vi "Ardwino-decifer-return.vi"(5 "Log file path":path=path "C:/Users/gsfcprime/Documents/Logs/FW_test-logs", 6 "New file?":bool, 7 "Reset history":bool, 8 "cycle  time":dbl, 9 "Switch query response":string, 10 "Responses history 2D in":string[][](array[string])=[["[Command Recv(18)]", "Motor ID     :", "State        :", "Direction    :", "Switch       :", "# of steps   :", "Step max rate:", "Ramp Slope   :", "# of position:", "com_success", "Q1S", "EOR1:"]], 11 "Arduino Response":string) -> (1 "Waveform Graph":dbl[][](graph), 2 "Responses history 2D out":string[][](array[string])=[["[Command Recv(18)]", "Motor ID     :", "State        :", "Direction    :", "Switch       :", "# of steps   :", "Step max rate:", "Ramp Slope   :", "# of position:", "com_success", "Q1S", "EOR1:"]], 3 "New  string to append":string[](array[string])=["[Command Recv(18)]", "Motor ID     :", "State        :", "Direction    :", "Switch       :", "# of steps   :", "Step max rate:", "Ramp Slope   :", "# of position:", "com_success", "Q1S", "EOR1:"], 4 "Log file out":path=path "C:/Users/gsfcprime/Documents/PRIME_documentation/FW_test_logs")   [LabVIEW 2021]
uses:
  <vilib>/Utility/file.llb/Write Delimited Spreadsheet (string).vi
  <vilib>/regexp/Match Regular Expression.xnode
panel:
  in  "(col) 2":i32=13
  out "Sw stae":u32(colorbox) caption="Sw state"
  out "after match":string
  out "before match":string
  out "m":i32
  out "substring":string
  in  "Motor #":string="0"
  in  "(col)":i32=12
  out "Array":dbl[](array[numeric])
  in  "List parameters":string[](array[string])=["[Command Recv(18)]", "Motor ID     :", "State        :", "Direction    :", "Switch       :", "# of steps   :", "Step max rate:", "Ramp Slope   :", "# of position:", "com_success", "Q1S", "EOR1:"]
  out "Ardwino responses -  Array":string[](array[string])=["[Command Recv(18)]", "Motor ID     :", "State        :", "Direction    :", "Switch       :", "# of steps   :", "Step max rate:", "Ramp Slope   :", "# of position:", "com_success", "Q1S", "EOR1:"]
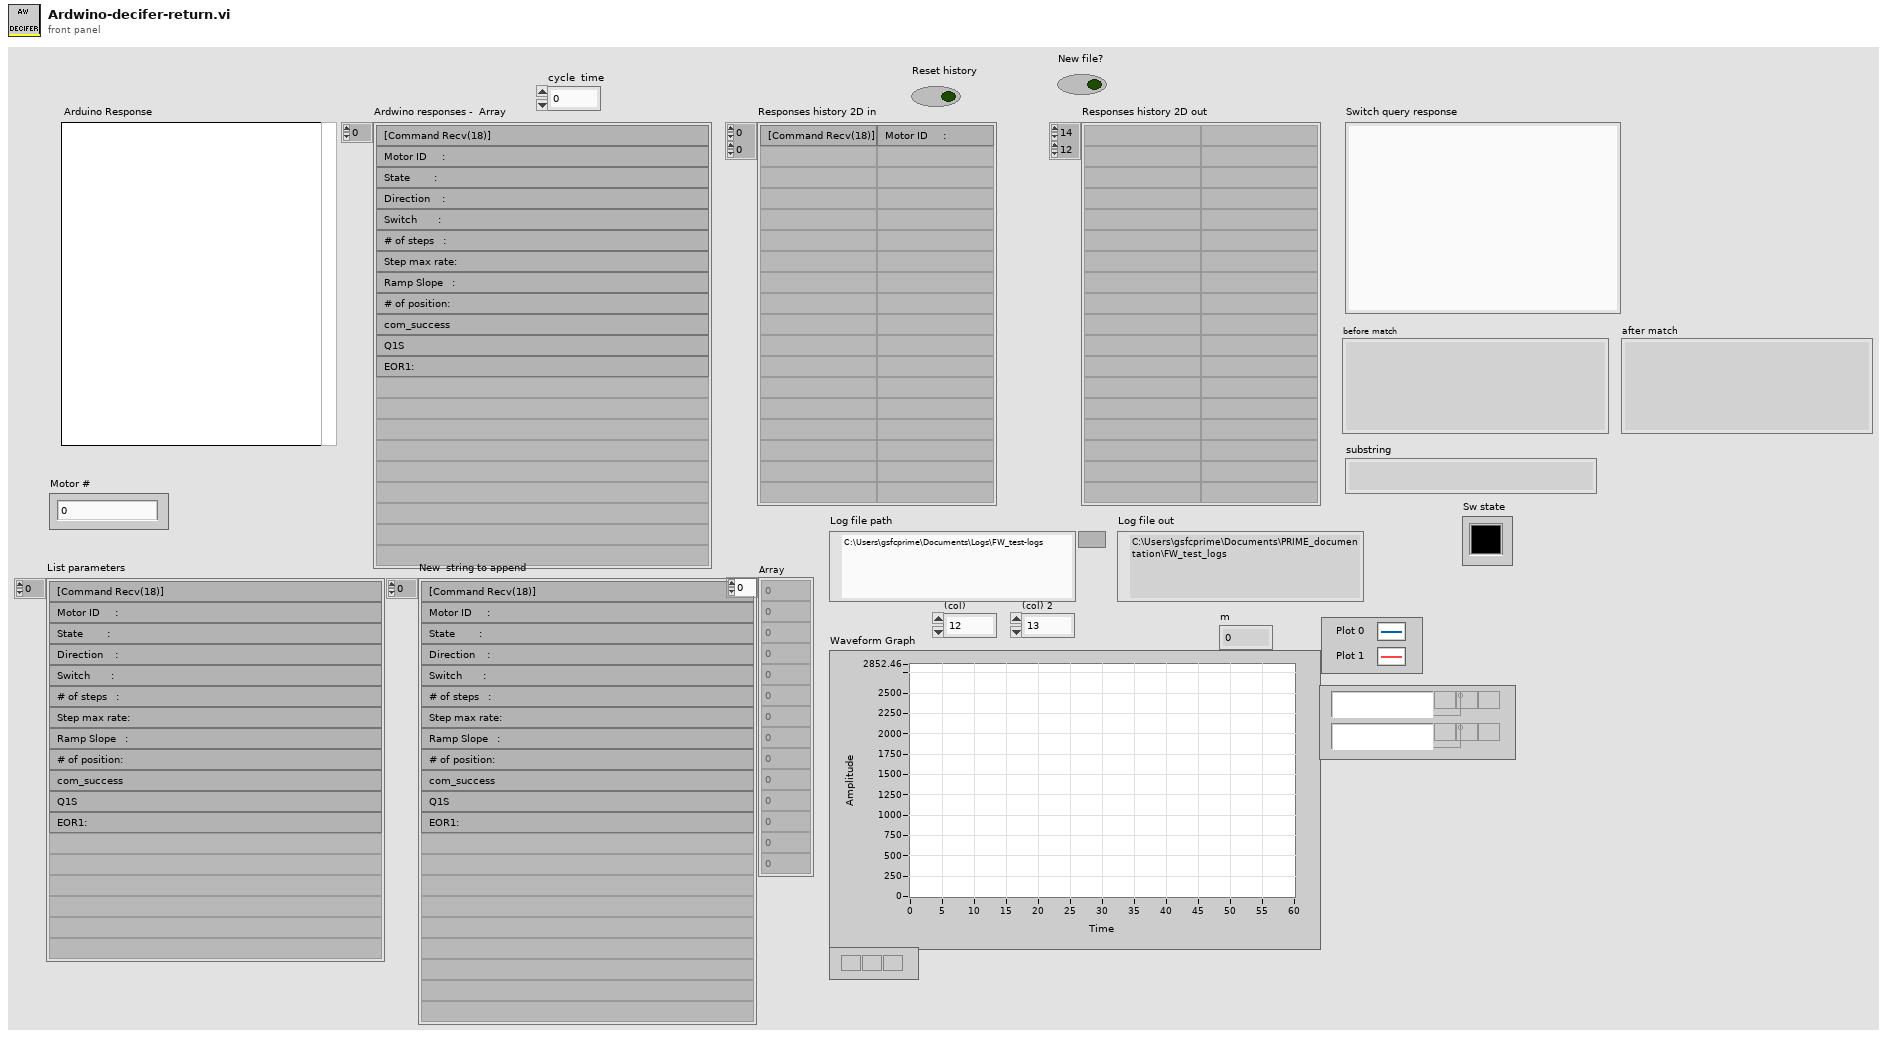
[diagram p1: front panel]
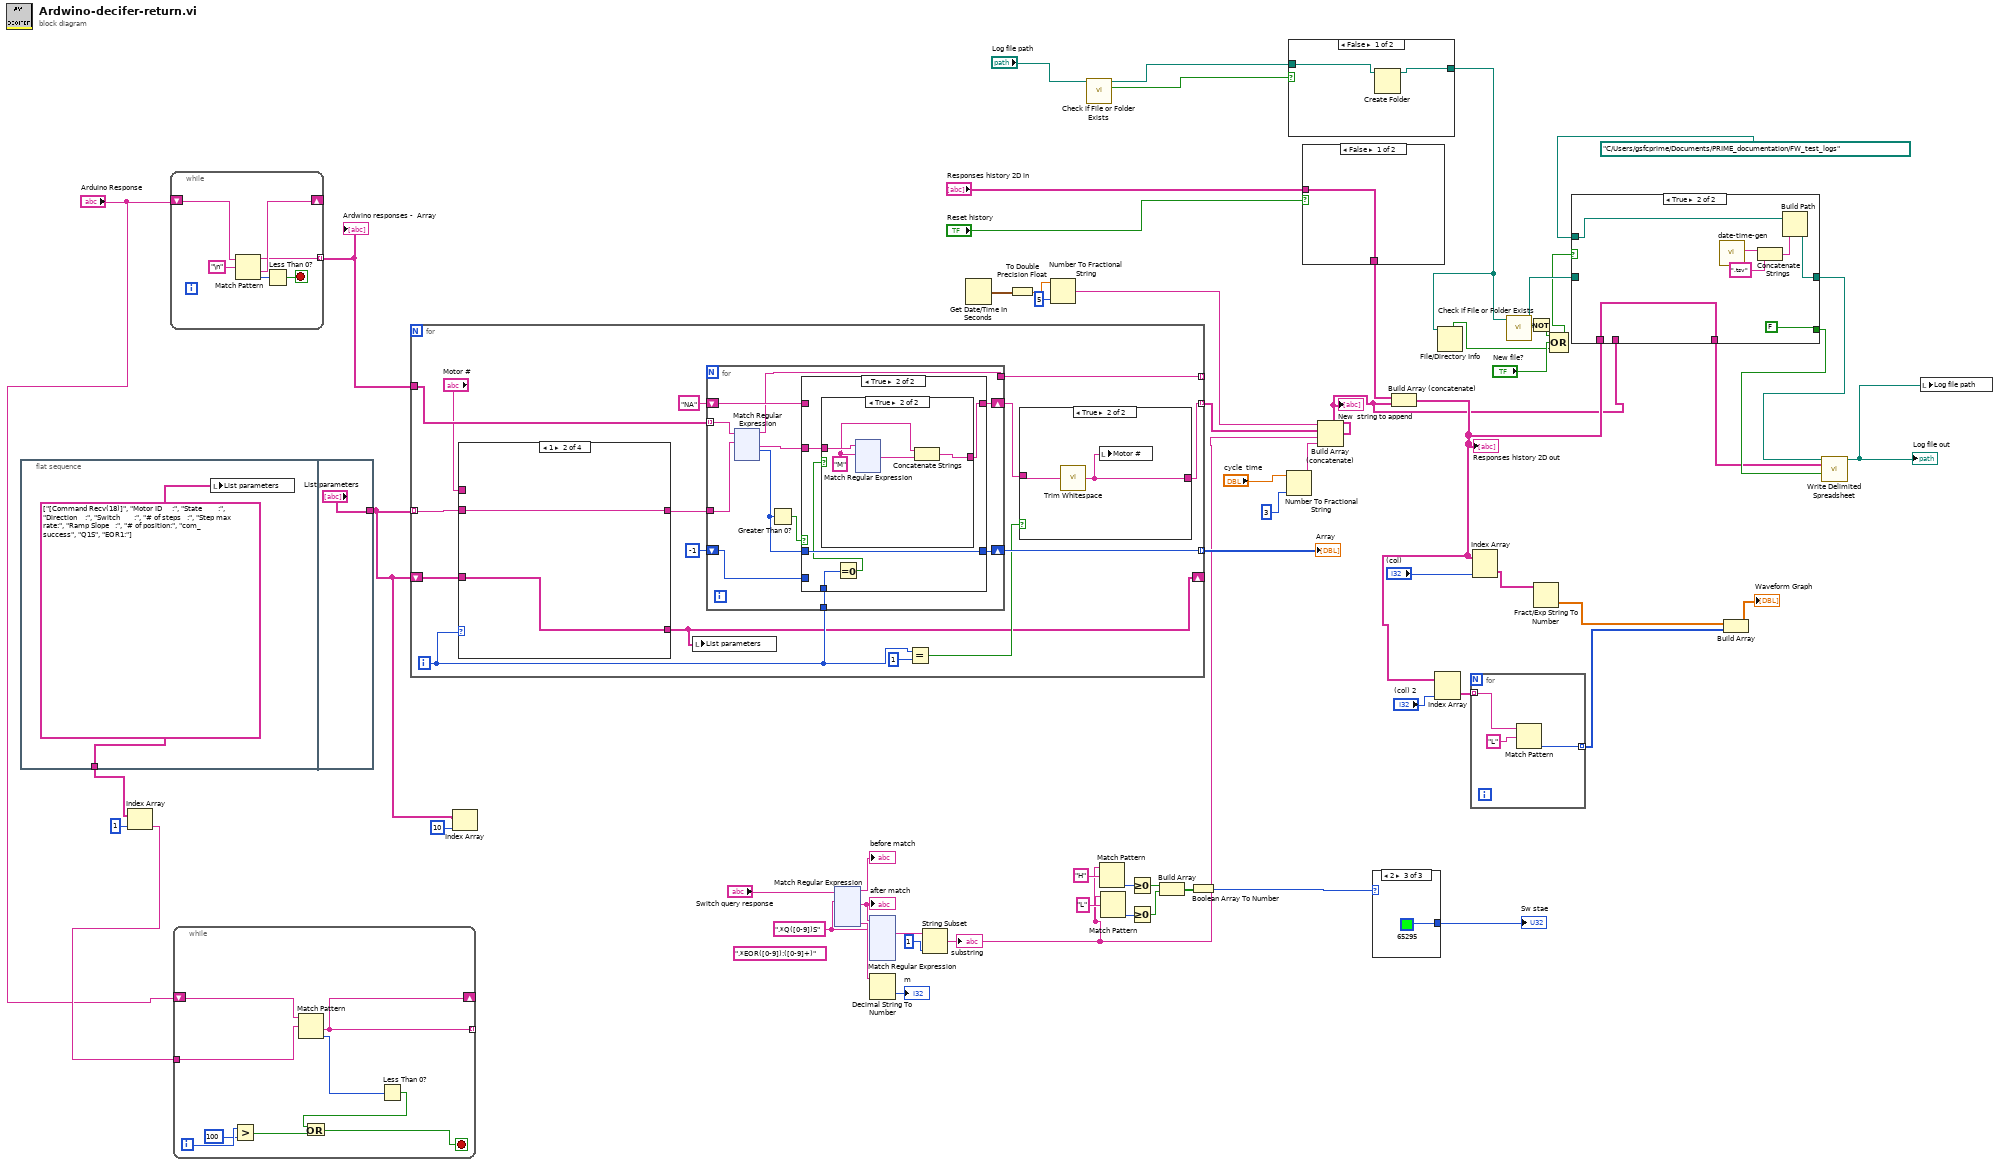
[diagram p0: block diagram]
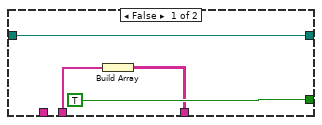
[diagram p3: hidden frame]
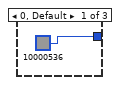
[diagram p4: hidden frame]
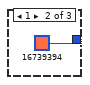
[diagram p5: hidden frame]
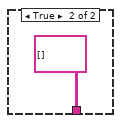
[diagram p6: hidden frame]
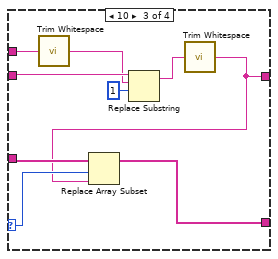
[diagram p8: hidden frame]
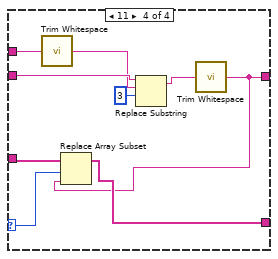
[diagram p9: hidden frame]
diagram:
  w43 = ".*Q([0-9])S" ("regular expression")
  (unwired) ".*EOR([0-9]):([0-9]+)" ("regular expression")
  n1 = flat-sequence {
    tunnel: [w62] -> w51
    tunnel: ["List parameters"] -> w55
    frame #0 {
      w62 = string[] ["[Command Recv(18)]", "Motor ID     :", "State        :", "Direction    :", "Switch       :", "# of steps   :", "Step max rate:", "Ramp Slope   :", "# of position:", "com_success", "Q1S", "EOR1:"] ("List parameters")
      n2 = local write "List parameters"(w62) -> ()
    }
    frame #1 {
    }
  }
  n3 = Index Array(array=w51, index=1) -> (element=w49:string)
  n4 = while {
    shift-right: [w68] -> _
    shift-left: "Arduino Response" -> [w69]
    tunnel: [w65] -> w52 mode=indexing
    stop <- w66 stop-if-true
    n5 = Match Pattern(string=w69, regular expression="\n") -> (before substring=w65:string, after substring=w68:string, offset past match=w67:i32)  [unwired: 1 in, 1 out]
    n6 = Less Than 0?(x=w67) -> (x < 0?=w66:bool)
  }
  "Ardwino responses -  Array" <- w52
  n7 = while {
    tunnel: w49 -> [w78]
    tunnel: [w75] -> _ mode=indexing
    shift-right: [w75] -> _
    shift-left: "Arduino Response" -> [w76]
    i -> [w73]
    stop <- w70 stop-if-true
    n8 = Greater?(x=w73, y=100) -> (0:w71:bool)
    n9 = Match Pattern(string=w76, regular expression=w78) -> (after substring=w75:string, offset past match=w77:i32)  [unwired: 1 in, 2 out]
    n10 = Less Than 0?(x=w77) -> (x < 0?=w74:bool)
    n11 = Or(x=w74, y=w71) -> (x .or. y?=w70:bool)
  }
  n12 = for {
    tunnel: w55 -> [w84] mode=indexing
    tunnel: w52 -> [w93]
    tunnel: [w81] -> w53 mode=indexing
    tunnel: [w90] -> w61 mode=indexing
    tunnel: [w89] -> _ mode=indexing
    shift-right: [w79] -> _
    shift-left: w55 -> [w80]
    i -> [w85]
    n13 = case shown="1" w85 {
      selector: w85 -> [_ _ w100 w111]
      tunnel: w84 -> [w95 w97 w106 w114]
      tunnel: "Motor #" -> [_ _ w105 w108]
      tunnel: [w95 w97 w98 w109] -> w82
      tunnel: w80 -> [w94 w96 w102 w113]
      tunnel: [w94 w96 w101 w112] -> w79
      frame 0, Default {
      }
      frame 1 {
      }
      frame 10 {
        n14 = call <vilib>:"Trim Whitespace.vi"("string"=w105) -> ("trimmed string"=w103:string)  [unwired: 1 in]
        n15 = Replace Substring(3:1 ("offset (0)"), 4:w103, 5:w106) -> (1:w99:string)  [unwired: 1 in, 1 out]
        n16 = call <vilib>:"Trim Whitespace.vi"("string"=w99) -> ("trimmed string"=w98:string)  [unwired: 1 in]
        n17 = Replace Array Subset(array=w102, new element=w98, index=w100) -> (w101:string[])
      }
      frame 11 {
        n18 = call <vilib>:"Trim Whitespace.vi"("string"=w108) -> ("trimmed string"=w107:string)  [unwired: 1 in]
        n19 = Replace Substring(3:3 ("offset (0)"), 4:w107, 5:w114) -> (1:w110:string)  [unwired: 1 in, 1 out]
        n20 = call <vilib>:"Trim Whitespace.vi"("string"=w110) -> ("trimmed string"=w109:string)  [unwired: 1 in]
        n21 = Replace Array Subset(array=w113, new element=w109, index=w111) -> (w112:string[])
      }
    }
    n22 = local write "List parameters"(w79) -> ()
    n23 = for {
      tunnel: w93 -> [w123] mode=indexing
      tunnel: w82 -> [w129]
      shift-right: [w121] -> w90
      shift-left: -1 ("offset past match") -> [w128]
      shift-right: [w127] -> w86
      shift-left: "NA" ("Arduino Responses") -> [w126]
      tunnel: [w120] -> w89
      tunnel: w85 -> [w119]
      n24 = xnode "Match Regular Expression"("input string"=w123, "regular expression"=w129) -> ("before match"=w120:string, "after match"=w125:string, "offset past match"=w122:i32)  [unwired: 4 in, 2 out]
      n25 = Greater Than 0?(x=w122) -> (x > 0?=w124:bool)
      n26 = case shown="True" w124 {
        tunnel: w128 -> [w247 _]
        tunnel: [w248 w249] -> w127
        tunnel: w126 -> [w248 _]
        tunnel: w125 -> [_ w250]
        tunnel: w122 -> [_ w253]
        tunnel: [w247 w253] -> w121
        tunnel: w119 -> [_ w252]
        frame False {
        }
        frame True {
          n27 = Equal To 0?(x=w252) -> (x = 0?=w251:bool)
          n28 = case shown="True" w251 {
            tunnel: w250 -> [w254 w258]
            tunnel: [w254 w256] -> w249
            frame False {
            }
            frame True {
              w255 = "M" ("regular expression")
              n29 = xnode "Match Regular Expression"("input string"=w258, "regular expression"=w255) -> ("after match"=w257:string)  [unwired: 4 in, 4 out]
              n30 = Concatenate Strings(w255, w257) -> (w256:string)
            }
          }
        }
      }
    }
    n31 = Equal?(x=w85, y=1) -> (x = y?=w87:bool)
    n32 = case shown="True" w87 {
      tunnel: w86 -> [w116 w118]
      tunnel: [w116 w117] -> w81
      frame False {
      }
      frame True {
        n33 = call <vilib>:"Trim Whitespace.vi"("string"=w118) -> ("trimmed string"=w117:string)  [unwired: 1 in]
        n34 = local write "Motor #"(w117) -> ()
      }
    }
  }
  "Array" <- w61
  n35 = Index Array(array=w55, index=10) -> ()  [unwired: 1 out]
  n36 = xnode "Match Regular Expression"("input string"="Switch query response", "regular expression"=w43) -> ("before match"=→"before match":string, "after match"=w44:string, "submatch 1"=w47:string)  [unwired: 4 in, 3 out]
  "after match" <- w44
  n37 = xnode "Match Regular Expression"("input string"=w44, "regular expression"=w43) -> ("after match"=w42:string)  [unwired: 4 in, 6 out]
  n38 = Decimal String To Number(string=w47) -> (number=→"m":i32)  [unwired: 2 in, 1 out]
  n39 = String Subset(string=w42, length (rest)=1 ("length (rest)")) -> (substring=w37:string)  [unwired: 1 in]
  "substring" <- w37
  n40 = Get Date/Time In Seconds() -> (seconds since 1Jan1904=w17:timestamp)
  n41 = To Double Precision Float(number=w17) -> (double precision float=w14:dbl)
  n42 = Number To Fractional String(number=w14, precision (6)=i16 5) -> (F-format string=w15:string)  [unwired: 2 in]
  n43 = call <vilib>:"Check if File or Folder Exists.vi"("path"="Log file path") -> ("file or folder exists?"=w4:bool, "dup path"=w5:path)  [unwired: 8 in, 1 out]
  n44 = Match Pattern(string=w37, regular expression="H") -> (offset past match=w36:i32)  [unwired: 1 in, 3 out]
  n45 = Match Pattern(string=w37, regular expression="L") -> (offset past match=w35:i32)  [unwired: 1 in, 3 out]
  n46 = Greater Or Equal To 0?(x=w36) -> (x >= 0?=w33:bool)
  n47 = Greater Or Equal To 0?(x=w35) -> (x >= 0?=w34:bool)
  n48 = Build Array(w33, w34) -> (w32:bool[])
  n49 = Boolean Array To Number(Boolean array=w32) -> (number=w31:u32)
  n50 = Number To Fractional String(number="cycle  time", precision (6)=i16 3) -> (F-format string=w1:string)  [unwired: 2 in]
  n51 = case shown="False" w4 {
    tunnel: w5 -> [w377 w378]
    tunnel: [w376 w378] -> w6
    frame False {
      n52 = Create Folder(path (use dialog)=w377) -> (created path=w376:path)  [unwired: 2 in, 2 out]
    }
    frame True {
    }
  }
  n53 = case shown="False" "Reset history" {
    tunnel: "Responses history 2D in" -> [w379 _]
    tunnel: [w379 string[][] [] ("Responses history 2D in")] -> w59
    frame False {
    }
    frame True {
    }
  }
  n54 = Build Array (concatenate)(w15, w53, w37, w1) -> (w10:string[])
  "New  string to append" <- w10
  n55 = case shown="2" w31 {
    tunnel: [u32 10000536 ("Color Box") u32 16739394 ("Color Box") u32 65295 ("Color Box")] -> w30
    frame 0, Default {
    }
    frame 1 {
    }
    frame 2 {
    }
  }
  "Sw stae" <- w30
  n56 = Build Array (concatenate)(w59, w10) -> (w12:string[][])
  "Responses history 2D out" <- w12
  n57 = Index Array(array=w12, index (col)="(col) 2") -> (element=w29:string[])  [unwired: 1 in]
  n58 = File/Directory Info(path=w6) -> (directory=w8:bool)  [unwired: 1 in, 6 out]
  n59 = for {
    tunnel: w29 -> [w386] mode=indexing
    tunnel: [w384] -> w28 mode=indexing
    n60 = Match Pattern(string=w386, regular expression="L") -> (offset past match=w384:i32)  [unwired: 1 in, 3 out]
  }
  n61 = Index Array(array=w12, index (col)="(col)") -> (element=w56:string[])  [unwired: 1 in]
  n62 = call <vilib>:"Check if File or Folder Exists.vi"("path"=w6) -> ("file or folder exists?"=w20:bool, "dup path"=w25:path)  [unwired: 8 in, 1 out]
  n63 = Not(x=w20) -> (.not. x?=w19:bool)
  n64 = Fract/Exp String To Number(string=w56) -> (number=w27:dbl[])  [unwired: 3 in, 1 out]
  n65 = Compound Arithmetic op=OR(w19, "New file?", w8) -> (w21:bool)
  n66 = case shown="True" w21 {
    tunnel: w25 -> [w390 _]
    tunnel: [w390 w392] -> w24
    tunnel: [TRUE FALSE] -> w23
    tunnel: path "C:/Users/gsfcprime/Documents/PRIME_documentation/FW_test_logs" ("Log file path") -> [_ w395]
    tunnel: w12 -> [_ w391]
    tunnel: [w387 w391] -> w11
    tunnel: w10 -> [w388 _]
    frame False {
      n67 = Build Array(w388) -> (w387:string[][])
    }
    frame True {
      n68 = call "date-time-gen.vi"() -> ("Date_time_string"=w396:string)  [unwired: 10 in, 1 out]
      n69 = Concatenate Strings(w396, ".tsv" ("string")) -> (w394:string)
      n70 = Build Path(base path=w395, name or relative path=w394) -> (appended path=w392:path)
    }
  }
  n71 = Build Array(w27, w28) -> (→"Waveform Graph":dbl[][])
  n72 = call-poly <vilib>:"Write Delimited Spreadsheet.vi"("file path (dialog if empty)"=w24, "2D data"=w11, "append to file? (new file:F)"=w23) -> ("new file path (Not A Path if cancelled)"=w13:path)  [unwired: 11 in, 1 out]
  "Log file out" <- w13
  n73 = local write "Log file path"(w13) -> ()
